vi "Set Tree Symbols All.vi"(8 "error in (no error)":errorcluster, 10 "symbol":i32, 11 "Tree Refnum":refnum<vi>) -> (0 "error out":errorcluster, 2 "Seted Tags":T1(array[cluster]), 3 "Tree Refnum":refnum<vi>)   [LabVIEW 2023, in "DSLV_Tree.lvlib"]
uses:
  DSLV_Tree.lvlib
panel:
  # "tips:\nsymbol num:symbol\n37:checkbox unselected\n38:checkbox selected"
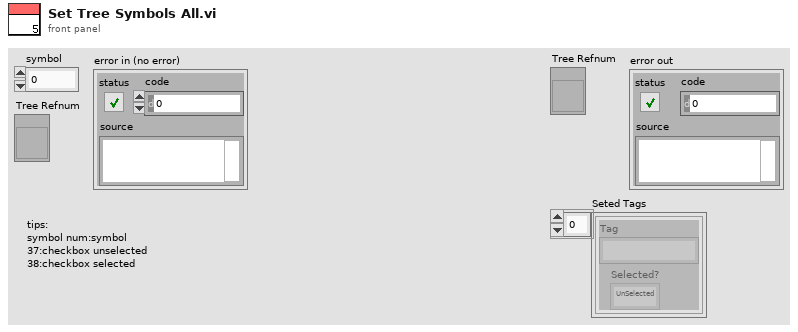
[diagram p1: front panel]
types:
  T1 = cluster{"Tag":string, "Selected?":enum16{"UnSelected", "Selected", "PartSelected"}}[]
  T2 = cluster{"Tag":string, "Selected?":enum16{"UnSelected", "Selected", "PartSelected"}}
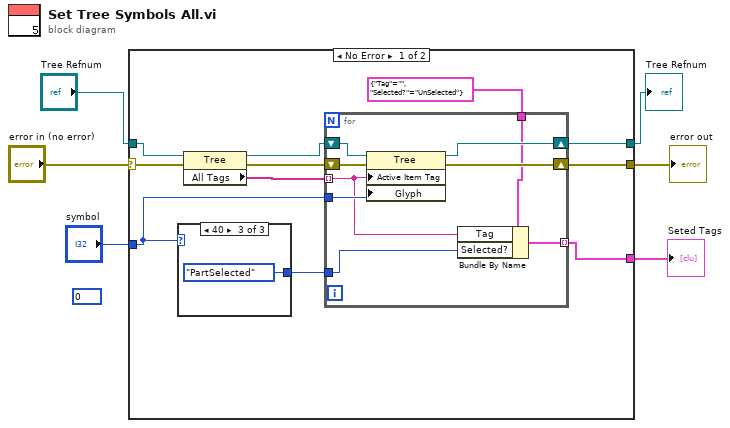
[diagram p0: block diagram]
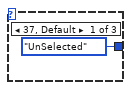
[diagram p2: hidden frame]
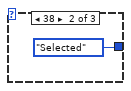
[diagram p3: hidden frame]
diagram:
  (unwired) 0
  n1 = case shown="No Error" "error in (no error)" {
    selector: "error in (no error)" -> [w13 w30]
    tunnel: "symbol" -> [w8 _]
    tunnel: [w15 w31] -> w5
    tunnel: "Tree Refnum" -> [w14 w31]
    tunnel: [w12 w30] -> w3
    tunnel: [w9 _] -> w1
    frame No Error {
      n2 = case shown="40" w8 {
        tunnel: [enum16{"UnSelected", "Selected", "PartSelected"}."UnSelected" ("Selected?") enum16{"UnSelected", "Selected", "PartSelected"}."Selected" ("Selected?") enum16{"UnSelected", "Selected", "PartSelected"}."PartSelected" ("Selected?")] -> w7
        frame 37, Default {
        }
        frame 38 {
        }
        frame 40 {
        }
      }
      n3 = property class="Tree"(reference=w14, error in=w13) -> (reference out=w16:refnum<vi>, error out=w17:errorcluster, "All Tags"=w11:string[])
      n4 = for {
        tunnel: w11 -> [w22] mode=indexing
        shift-right: [w26] -> w12
        shift-left: w17 -> [w28]
        shift-right: [w27] -> w15
        shift-left: w16 -> [w29]
        tunnel: w8 -> [w25]
        tunnel: T2 {"Tag"="", "Selected?"=enum."UnSelected"} ("Set") -> [w24]
        tunnel: [w23] -> w9 mode=indexing
        tunnel: w7 -> [w21]
        n5 = property on="Property Node" class="Tree"(reference=w29, error in=w28, "Active Item Tag"=w22, "Glyph"=w25) -> (reference out=w27:refnum<vi>, error out=w26:errorcluster)
        n6 = Bundle By Name(cluster=w24, "Tag"=w22, "Selected?"=w21) -> (w23:T2)
      }
    }
    frame Error {
    }
  }
  "Tree Refnum" <- w5
  "error out" <- w3
  "Seted Tags" <- w1
